vi "Draw.vi"(0 "FSM.Edge In":refnum<class "FSM.Edge.lvclass">, 7 "picture in":picture, 11 "selected":bool) -> (4 "FSM.Edge Out":refnum<class "FSM.Edge.lvclass">, 8 "picture out":picture)   [LabVIEW 2020, in "FSM.Edge.lvclass"]
uses:
  FSM.Edge.lvclass
  FSM.Edge.lvclass/FSM.Edge.ctl
  FSM.Label/FSM.Label.lvclass/FSM.Label.ctl
  FSM.Label/Read rect.vi
  FSM.Label/FSM.Label.lvclass
  FSM.Annotation/FSM.Annotation.lvclass
panel:
  out "error out":errorcluster
  in  "error in (no error)":errorcluster
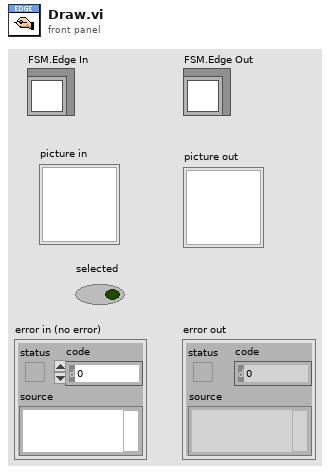
[diagram p1: front panel]
types:
  T1 = cluster{"Width":u16, "Style":enum32{"Solid", "Dash", "Dot", "DashDot", "DashDotDot"}}
  T2 = enum32{"Solid", "Dash", "Dot", "DashDot", "DashDotDot"}
  T3 = cluster{"left":i16, "top":i16, "right":i16, "bottom":i16}
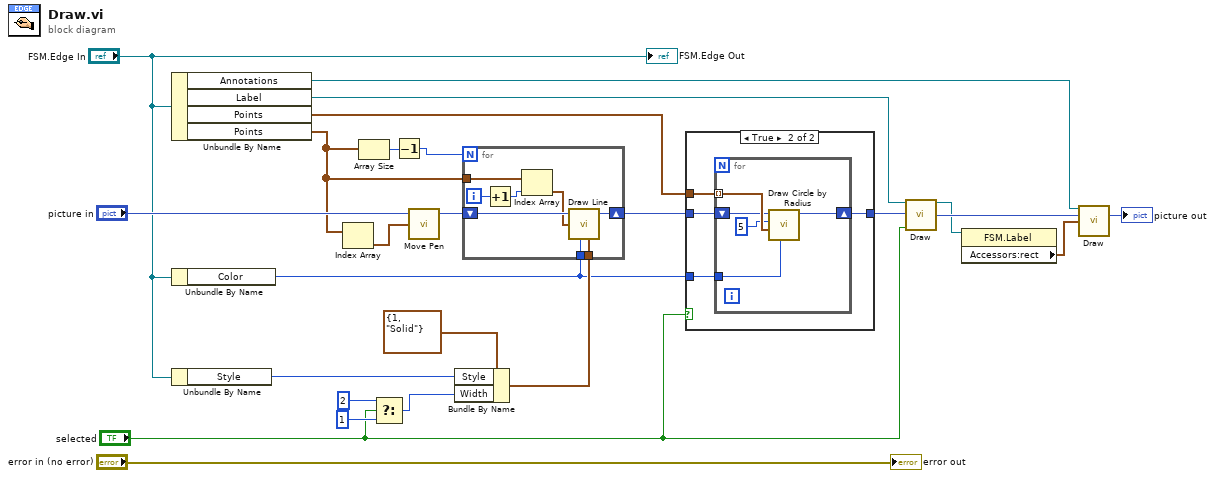
[diagram p0: block diagram]
diagram:
  n1 = Unbundle By Name("FSM.Edge In") -> ("Annotations"=w5:refnum<class "FSM.Annotation.lvclass">, "Label"=w17:refnum<class "FSM.Label.lvclass">, "Points"=w4:cluster{"x":i16, "y":i16}[], "Points"=w8:cluster{"x":i16, "y":i16}[])
  n2 = Unbundle By Name("FSM.Edge In") -> ("Color"=w11:u32)
  n3 = Unbundle By Name("FSM.Edge In") -> ("Style"=w18:T2)
  n4 = Index Array(array=w8) -> (element=w24:cluster{"x":i16, "y":i16})  [unwired: 1 in]
  n5 = Array Size(array=w8) -> (size(s)=w10:i32)
  n6 = Select(t=2, s="selected", f=1) -> (s? t:f=w15:i32)
  n7 = Decrement(x=w10) -> (x-1=w9:i32)
  n8 = call <vilib>:"Move Pen.vi"("new position"=w24, "picture"="picture in") -> ("new picture"=w23:picture)  [unwired: 3 in]
  n9 = Bundle By Name(cluster=T1 {"Width"=1, "Style"=enum."Solid"} ("pen"), "Style"=w18, "Width"=w15) -> (w20:T1)
  n10 = for {
    N: w9 -> [_]
    tunnel: w20 -> [w32]
    tunnel: w11 -> [w30]
    shift-right: [w31] -> w13
    shift-left: w23 -> [w33]
    tunnel: w8 -> [w29]
    i -> [w27]
    n11 = Increment(x=w27) -> (x+1=w26:i32)
    n12 = Index Array(array=w29, index=w26) -> (element=w28:cluster{"x":i16, "y":i16})
    n13 = call <vilib>:"Draw Line.vi"("picture"=w33, "end point"=w28, "color(black)"=w30, "pen"=w32) -> ("new picture"=w31:picture)  [unwired: 5 in]
  }
  n14 = case shown="True" "selected" {
    tunnel: w13 -> [w34 w38]
    tunnel: [w34 w37] -> w12
    tunnel: w4 -> [_ w36]
    tunnel: w11 -> [_ w35]
    frame False {
    }
    frame True {
      n15 = for {
        shift-right: [w41] -> w37
        shift-left: w38 -> [w42]
        tunnel: w36 -> [w43] mode=indexing
        tunnel: w35 -> [w39]
        n16 = call <vilib>:"Draw Circle by Radius.vi"("color(black)"=w39, "pixel center"=w43, "radius"=i16 5, "picture"=w42) -> ("new picture"=w41:picture)  [unwired: 7 in]
      }
    }
  }
  n17 = call "Draw.vi"("FSM.Label"=w17, "picture in"=w12, "selected"="selected") -> ("FSM.Label thru"=w2:refnum<class "FSM.Label.lvclass">, "picture out"=w7:picture)  [unwired: 11 in]
  n18 = property class="FSM.Label"(reference=w2) -> ("Accessors:rect"=w1:T3)  [unwired: 1 in, 2 out]
  n19 = call "Draw.vi"("FSM.Annotation in"=w5, "picture in"=w7, "Label rect"=w1) -> ("picture out"=→"picture out":picture)  [unwired: 10 in, 2 out]
  "FSM.Edge Out" <- "FSM.Edge In"
  "error out" <- "error in (no error)"
